vi "parse HarpMessage.vi"(13 "Round value":bool) -> (4 "HarpDataFrame":T1={"Timestamp(us)"=0.0, "Command"=16, "Error"=FALSE, "Register Address"=16, "Port"=16, "Number of Elements"=16, "Type"=16, "I8"=0, "U8"=0, "U16"=0, "I16"=0, "U32"=0, "I32"=0, "U64"=0, "I64"=0, "Float"=0.0, "U8[]"=[], "I8[]"=[], "U16[]"=[], "I16[]"=[], "U32[]"=[], "I32[]"=[], "U64[]"=[], "I64[]"=[], "Float[]"=[]} {"Timestamp(us)" format="%.6f"}, 8 "Packet Found":bool, 15 "Byte Rejected":bool)   [LabVIEW 2010]
panel:
  out "Float[]":sgl[](array[numeric])
  out "I64[]":i64[](array[numeric])
  out "U64[]":u64[](array[numeric])
  out "I32[]":i32[](array[numeric])
  out "U32[]":u32[](array[numeric])
  out "I16[]":i16[](array[numeric])
  out "U16[]":u16[](array[numeric])
  out "I8[]":i8[](array[numeric])
  out "U8[]":u8[](array[numeric])
  out "Float":sgl
  out "I64":i64
  out "U64":u64
  out "I32":i32
  out "U32":u32
  out "I16":i16
  out "U16":u16
  out "U8":u8
  out "I8":i8
  in  "Enum":T2(ring)
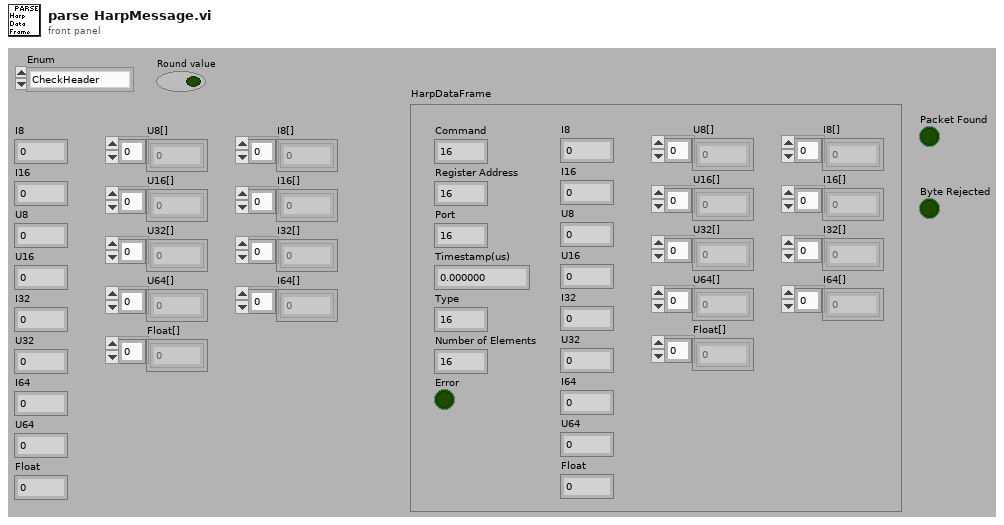
[diagram p1: front panel]
types:
  T1 = cluster{"Timestamp(us)":dbl, "Command":u8, "Error":bool, "Register Address":u8, "Port":u8, "Number of Elements":u8, "Type":u8, "I8":i8, "U8":u8, "U16":u16, "I16":i16, "U32":u32, "I32":i32, "U64":u64, "I64":i64, "Float":sgl, "U8[]":u8[], "I8[]":i8[], "U16[]":u16[], "I16[]":i16[], "U32[]":u32[], "I32[]":i32[], "U64[]":u64[], "I64[]":i64[], "Float[]":sgl[]}
  T2 = enum16{"CheckHeader", "CheckChekcum", "Parse", "Exit"}
  T3 = enum16{"CreateBuffer", "WriteBytes", "WriteByte", "AvailableMemory", "OccupiedMemory", "CheckBytes", "ReadBytes"}
  T4 = enum16{"big-endian, network order", "native, host order", "little-endian"}
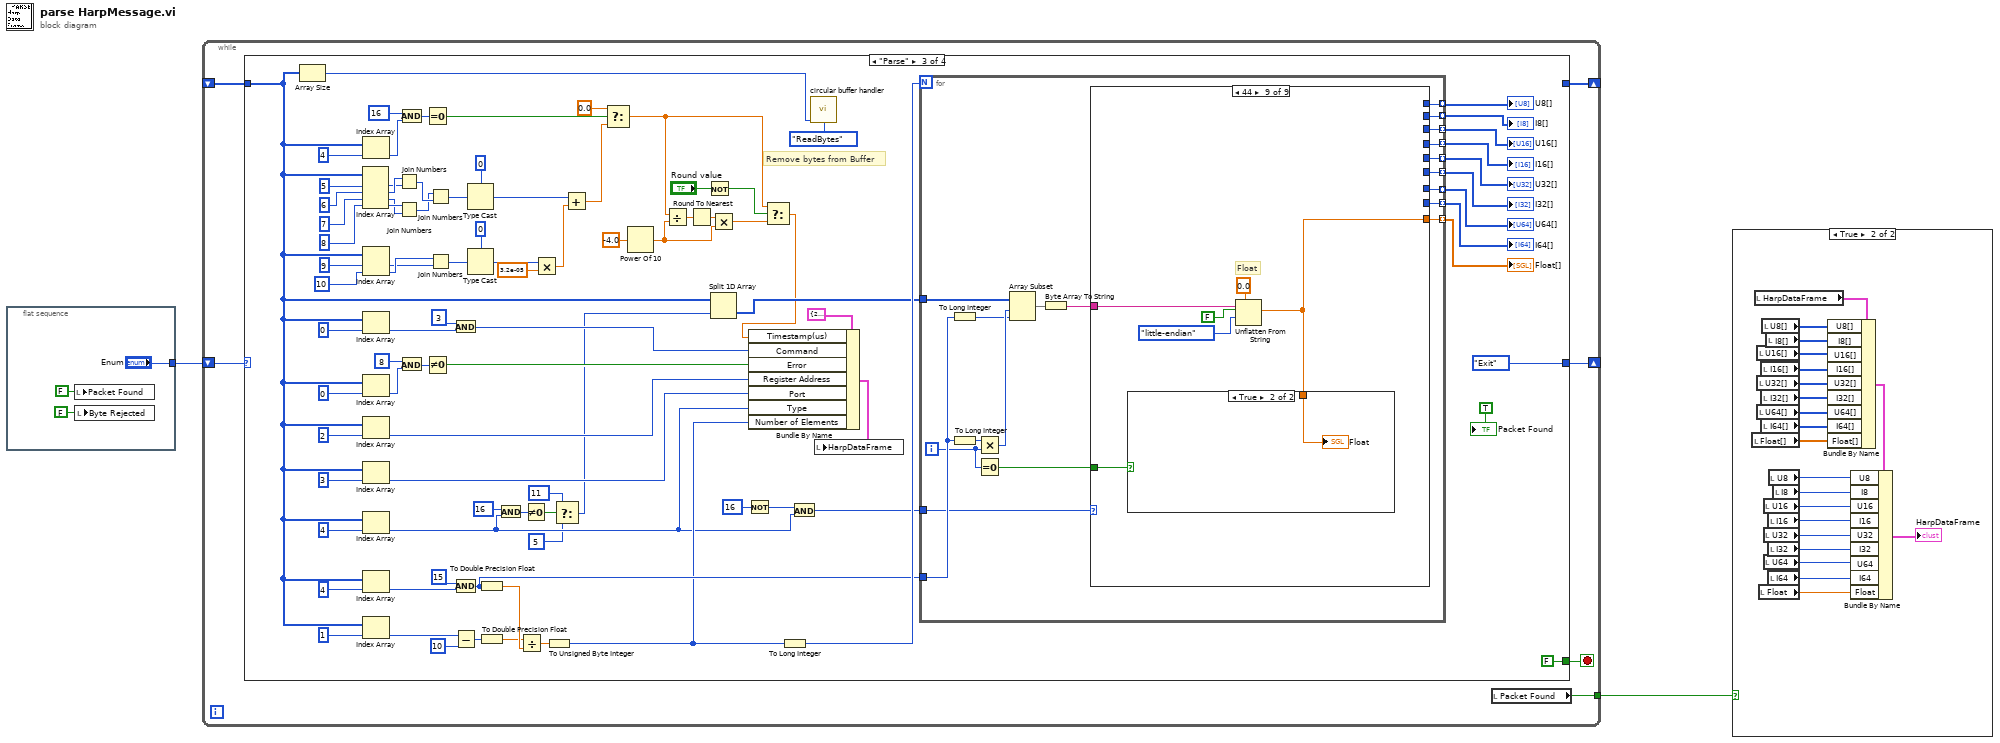
[diagram p0: block diagram]
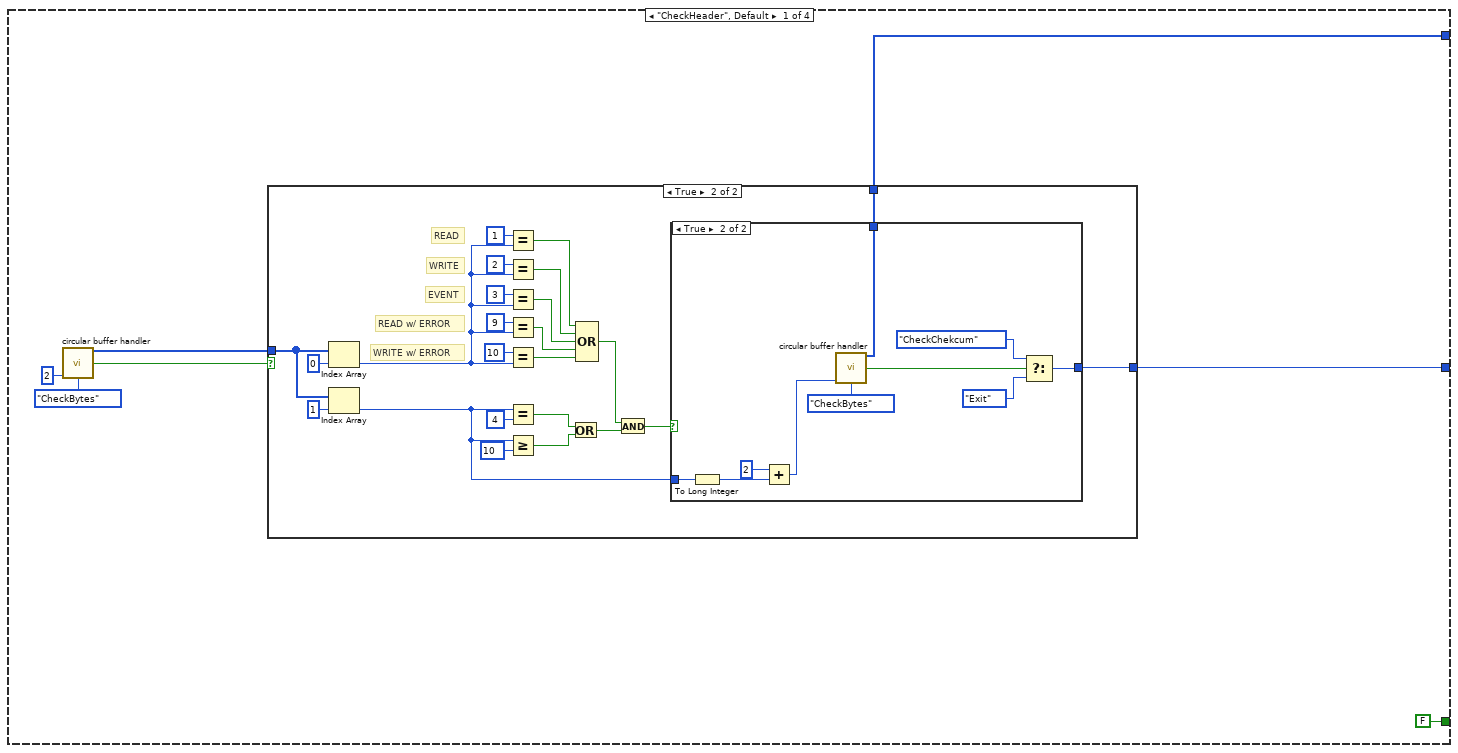
[diagram p3: hidden frame]
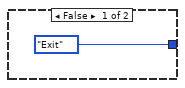
[diagram p4: hidden frame]
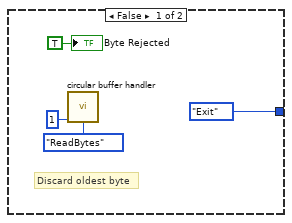
[diagram p5: hidden frame]
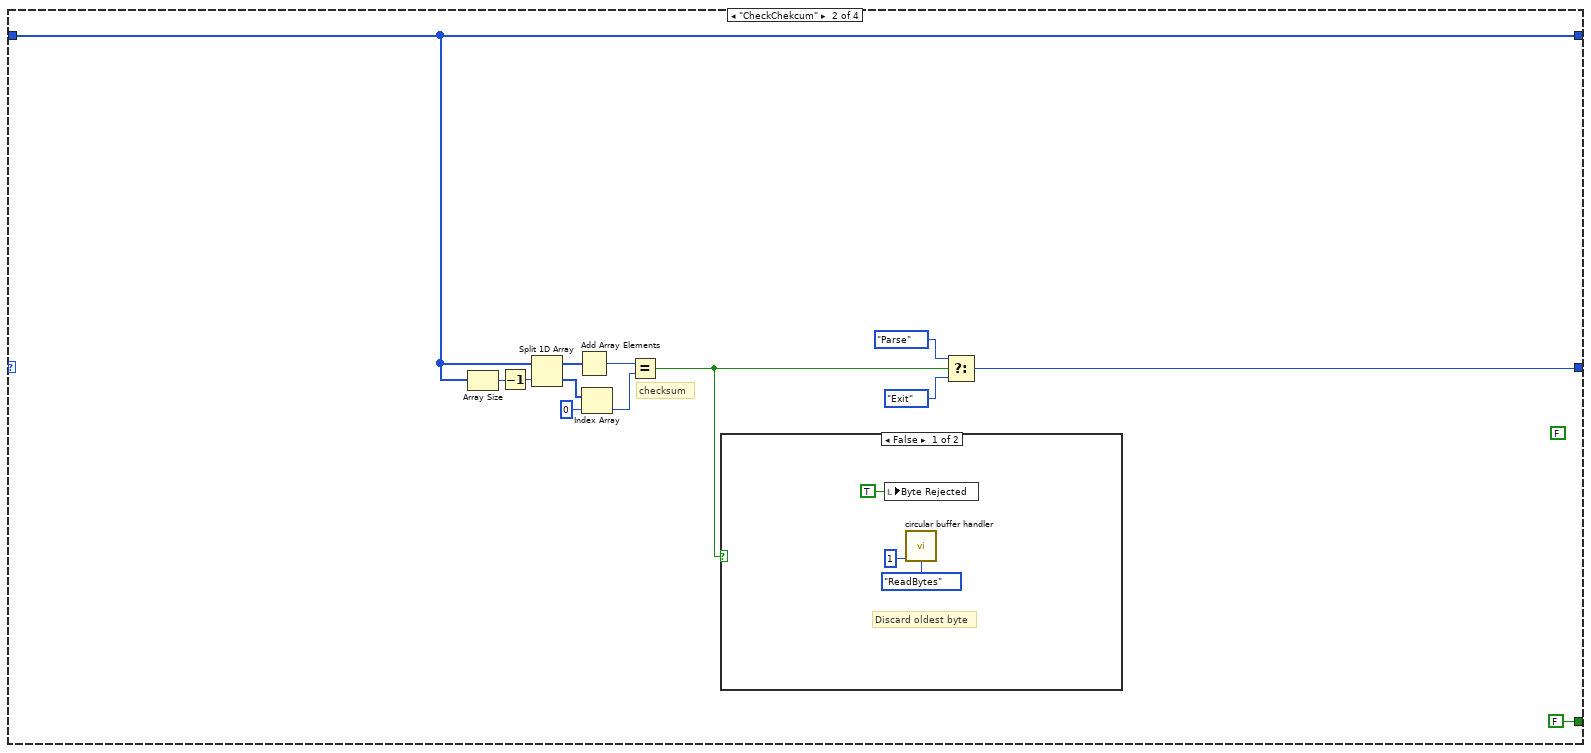
[diagram p6: hidden frame]
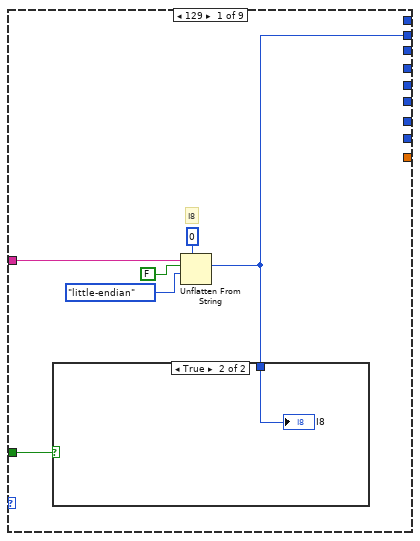
[diagram p8: hidden frame]
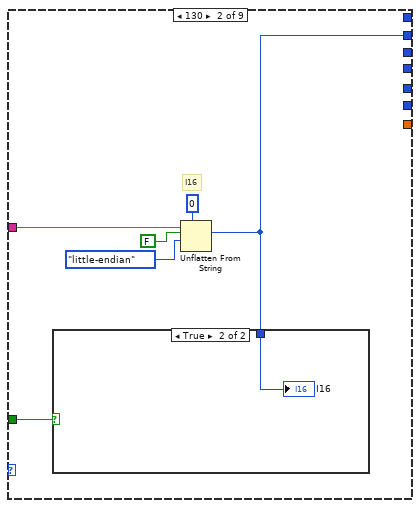
[diagram p10: hidden frame]
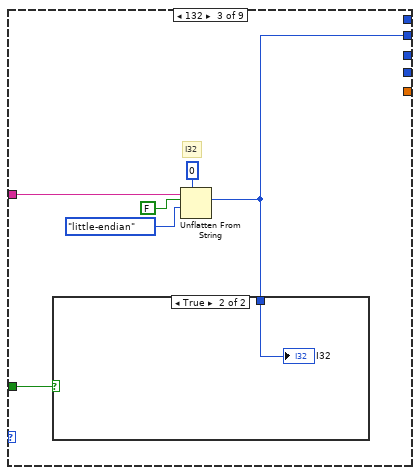
[diagram p12: hidden frame]
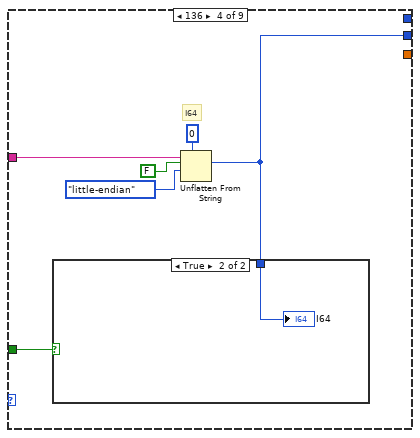
[diagram p14: hidden frame]
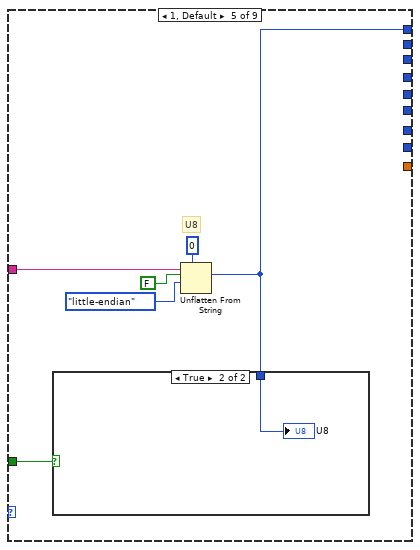
[diagram p16: hidden frame]
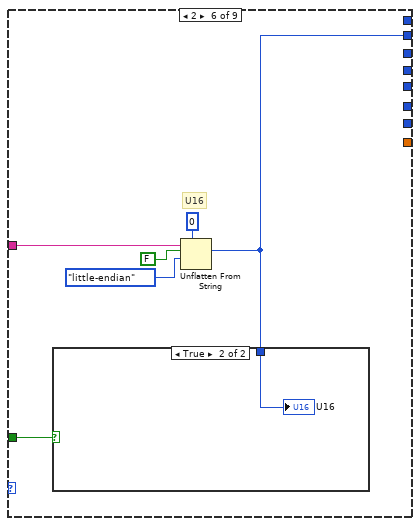
[diagram p18: hidden frame]
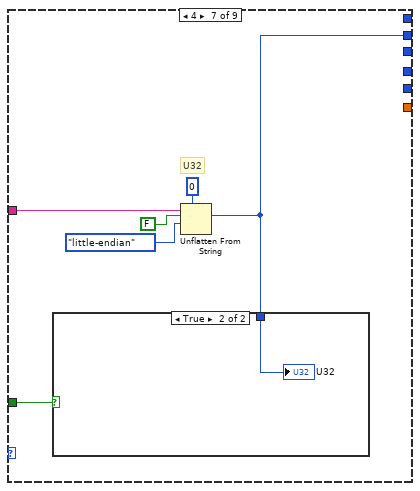
[diagram p20: hidden frame]
diagram:
  n1 = flat-sequence {
    tunnel: ["Enum"] -> w2
    frame #0 {
      n2 = local write "Packet Found"(FALSE ("PacketFound")) -> ()
      n3 = local write "Byte Rejected"(FALSE ("Byte Rejected")) -> ()
    }
  }
  n4 = while {
    shift-right: [w10] -> _
    shift-left: w2 -> [w11]
    shift-right: [w9] -> _
    shift-left: _ -> [w8]
    tunnel: [w6] -> w1
    stop <- w7 stop-if-true
    n5 = case shown="\"Parse\"" w11 {
      tunnel: [w14 w61 T2."Exit" ("Enum") T2."Exit" ("Enum")] -> w10
      tunnel: [w13 w58 _ _] -> w9
      tunnel: w8 -> [_ w58 w113 _]
      tunnel: [FALSE FALSE FALSE TRUE] -> w7
      frame "CheckHeader", Default {
        n6 = call "circular buffer handler.vi"("NumberOfBytes"=2, "Enum"=T3."CheckBytes") -> ("OutputBytes"=w15:u8[], "OK"=w16:bool)  [unwired: 11 in, 1 out]
        n7 = case shown="True" w16 {
          tunnel: w15 -> [_ w41]
          tunnel: [T2."Exit" ("Enum") w21] -> w14
          tunnel: [_ w20] -> w13
          frame False {
          }
          frame True {
            # "WRITE w/ ERROR"
            # "READ w/ ERROR"
            # "EVENT"
            # "WRITE"
            # "READ"
            n8 = Index Array(array=w41, index=0) -> (element=w35:u8)
            n9 = Index Array(array=w41, index=1) -> (element=w22:u8)
            n10 = Equal?(x=u8 1, y=w35) -> (x = y?=w34:bool)
            n11 = Equal?(x=u8 2, y=w35) -> (x = y?=w33:bool)
            n12 = Equal?(x=u8 3, y=w35) -> (x = y?=w32:bool)
            n13 = Equal?(x=u8 9, y=w35) -> (x = y?=w31:bool)
            n14 = Equal?(x=u8 10, y=w35) -> (x = y?=w30:bool)
            n15 = Equal?(x=w22, y=u8 4 ("x")) -> (x = y?=w27:bool)
            n16 = Greater Or Equal?(x=w22, y=u8 10 ("x")) -> (x >= y?=w26:bool)
            n17 = Or(x=w27, y=w26) -> (x .or. y?=w25:bool)
            n18 = Compound Arithmetic op=OR(w34, w33, w32, w31, w30) -> (w24:bool)
            n19 = And(x=w24, y=w25) -> (x .and. y?=w23:bool)
            n20 = case shown="True" w23 {
              tunnel: w22 -> [_ w56]
              tunnel: [T2."Exit" ("Enum") w53] -> w21
              tunnel: [_ w48] -> w20
              frame False {
                # "Discard oldest byte"
                n21 = call "circular buffer handler.vi"("NumberOfBytes"=1, "Enum"=T3."ReadBytes") -> ()  [unwired: 11 in, 3 out]
                "Byte Rejected" <- TRUE ("PacketFound")
              }
              frame True {
                n22 = To Long Integer(number=w56) -> (32bit integer=w54:i32)
                n23 = Add(x=2, y=w54) -> (x+y=w50:i32)
                n24 = call "circular buffer handler.vi"("NumberOfBytes"=w50, "Enum"=T3."CheckBytes") -> ("OutputBytes"=w48:u8[], "OK"=w49:bool)  [unwired: 11 in, 1 out]
                n25 = Select(t=T2."CheckChekcum" ("Enum"), s=w49, f=T2."Exit" ("Enum")) -> (s? t:f=w53:T2)
              }
            }
          }
        }
      }
      frame "CheckChekcum" {
        (unwired) FALSE ("PacketFound")
        # "checksum"
        n26 = Array Size(array=w58) -> (size(s)=w70:i32)
        n27 = Decrement(x=w70) -> (x-1=w69:i32)
        n28 = Split 1D Array(array=w58, index=w69) -> (first subarray=w65:u8[], second subarray=w66:u8[])
        n29 = Add Array Elements(numeric array=w65) -> (sum=w68:u8)
        n30 = Index Array(array=w66, index=0) -> (element=w64:u8)
        n31 = Equal?(x=w68, y=w64) -> (x = y?=w59:bool)
        n32 = case shown="False" w59 {
          frame False {
            # "Discard oldest byte"
            n33 = local write "Byte Rejected"(TRUE ("Byte Rejected")) -> ()
            n34 = call "circular buffer handler.vi"("NumberOfBytes"=1, "Enum"=T3."ReadBytes") -> ()  [unwired: 11 in, 3 out]
          }
          frame True {
          }
        }
        n35 = Select(t=T2."Parse" ("Enum"), s=w59, f=T2."Exit" ("Enum")) -> (s? t:f=w61:T2)
      }
      frame "Parse" {
        # "Remove bytes from Buffer"
        n36 = Array Size(array=w113) -> (size(s)=w115:i32)
        n37 = Index Array(array=w113, index #1=5 ("index"), index #2=6 ("index"), index #3=7 ("index"), index #4=8 ("index")) -> (element #1=w155:u8, element #2=w159:u8, element #3=w156:u8, element #4=w157:u8)
        n38 = Index Array(array=w113, index=4) -> (element=w140:u8)
        n39 = Index Array(array=w113, index #1=9 ("index"), index #2=10 ("index")) -> (element #1=w144:u8, element #2=w145:u8)
        n40 = Index Array(array=w113, index=0) -> (element=w134:u8)
        n41 = Index Array(array=w113, index=0) -> (element=w133:u8)
        n42 = Index Array(array=w113, index=2) -> (element=w99:u8)
        n43 = Index Array(array=w113, index=3) -> (element=w98:u8)
        n44 = Index Array(array=w113, index=4) -> (element=w89:u8)
        n45 = Index Array(array=w113, index=4) -> (element=w126:u8)
        n46 = Index Array(array=w113, index=1) -> (element=w122:u8)
        n47 = Join Numbers(hi=w159, lo=w155) -> ((hi.lo)=w160:u16)
        n48 = Join Numbers(hi=w157, lo=w156) -> ((hi.lo)=w158:u16)
        n49 = And(x=u8 16, y=w140) -> (x .and. y?=w164:u8)
        n50 = And(x=u8 8, y=w133) -> (x .and. y?=w131:u8)
        n51 = Equal To 0?(x=w164) -> (x = 0?=w139:bool)
        n52 = Not Equal To 0?(x=w131) -> (x != 0?=w100:bool)
        n53 = Join Numbers(hi=w158, lo=w160) -> ((hi.lo)=w150:u32)
        n54 = Join Numbers(hi=w145, lo=w144) -> ((hi.lo)=w146:u16)
        n55 = And(x=u8 3, y=w134) -> (x .and. y?=w101:u8)
        n56 = And(x=u8 15, y=w126) -> (x .and. y?=w111:u8)
        n57 = Subtract(x=w122, y=u8 10) -> (x-y=w120:u8)
        n58 = Type Cast(type=u32 0 ("byte count"), x=w150) -> (*(type *) &x=w162:u32)
        n59 = Type Cast(type=u16 0 ("byte count"), x=w146) -> (*(type *) &x=w148:u16)
        n60 = To Double Precision Float(number=w111) -> (double precision float=w118:dbl)
        n61 = To Double Precision Float(number=w120) -> (double precision float=w117:dbl)
        n62 = And(x=u8 16, y=w89) -> (x .and. y?=w90:u8)
        n63 = Divide(x=w117, y=w118) -> (x/y=w119:dbl)
        n64 = Not Equal To 0?(x=w90) -> (x != 0?=w88:bool)
        n65 = Multiply(x=w148, y=3.2e-05) -> (x*y=w163:dbl)
        n66 = To Unsigned Byte Integer(number=w119) -> (unsigned 8bit integer=w97:u8)
        n67 = Select(t=u8 11, s=w88, f=u8 5) -> (s? t:f=w85:u8)
        n68 = Add(x=w162, y=w163) -> (x+y=w138:dbl)
        n69 = Select(t=0.0, s=w139, f=w138) -> (s? t:f=w77:dbl)
        n70 = Power Of 10(x=-4.0) -> (10^x=w80:dbl)
        n71 = Divide(x=w77, y=w80) -> (x/y=w82:dbl)
        n72 = Round To Nearest(number=w82) -> (nearest integer value=w81:dbl)
        n73 = Not(x="Round value") -> (.not. x?=w74:bool)
        n74 = Multiply(x=w81, y=w80) -> (x*y=w78:dbl)
        n75 = Split 1D Array(array=w113, index=w85) -> (second subarray=w92:u8[])  [unwired: 1 out]
        n76 = Not(x=u8 16) -> (.not. x?=w95:u8)
        n77 = Select(t=w77, s=w74, f=w78) -> (s? t:f=w76:dbl)
        n78 = Bundle By Name(cluster=T1 {"Timestamp(us)"=2218.246816, "Command"=1, "Error"=FALSE, "Register Address"=18, "Port"=255, "Number of Elements"=1, "Type"=84, "I8"=0, "U8"=0, "U16"=0, "I16"=0, "U32"=0, "I32"=0, "U64"=0, "I64"=0, "Float"=0.0, "U8[]"=[0], "I8[]"=[0], "U16[]"=[0], "I16[]"=[0], "U32[]"=[0], "I32[]"=[0], "U64[]"=[0], "I64[]"=[0], "Float[]"=[0.0]} ("HarpDataFrame"), "Timestamp(us)"=w76, "Command"=w101, "Error"=w100, "Register Address"=w99, "Port"=w98, "Type"=w89, "Number of Elements"=w97) -> (w84:T1)
        n79 = To Long Integer(number=w97) -> (32bit integer=w112:i32)
        n80 = And(x=w95, y=w89) -> (x .and. y?=w93:u8)
        n81 = call "circular buffer handler.vi"("NumberOfBytes"=w115, "Enum"=T3."ReadBytes") -> ()  [unwired: 11 in, 3 out]
        n82 = local write "HarpDataFrame"(w84) -> ()
        n83 = for {
          N: w112 -> [_]
          tunnel: w92 -> [w183]
          tunnel: w111 -> [w182]
          tunnel: w93 -> [w178]
          tunnel: [w175] -> w110 mode=indexing
          tunnel: [w174] -> w109 mode=indexing
          tunnel: [w173] -> w108 mode=indexing
          tunnel: [w172] -> w107 mode=indexing
          tunnel: [w171] -> w106 mode=indexing
          tunnel: [w170] -> w105 mode=indexing
          tunnel: [w169] -> w104 mode=indexing
          tunnel: [w168] -> w102 mode=indexing
          tunnel: [w167] -> w103 mode=indexing
          i -> [w177]
          n84 = To Long Integer(number=w182) -> (32bit integer=w179:i32)
          n85 = To Long Integer(number=w182) -> (32bit integer=w180:i32)
          n86 = Multiply(x=w180, y=w177) -> (x*y=w181:i32)
          n87 = Equal To 0?(x=w177) -> (x = 0?=w176:bool)
          n88 = Array Subset(array=w183, index=w181, length=w179) -> (w184:u8[])
          n89 = Byte Array To String(unsigned byte array=w184) -> (string=w185:string)
          n90 = case shown="44" w178 {
            tunnel: w185 -> [w190 w197 w204 w211 w218 w225 w232 w239 w246]
            tunnel: w176 -> [w187 w194 w201 w208 w215 w222 w229 w236 w243]
            tunnel: [_ _ _ _ w214 _ _ _ _] -> w175
            tunnel: [w186 _ _ _ _ _ _ _ _] -> w174
            tunnel: [_ _ _ _ _ w221 _ _ _] -> w173
            tunnel: [_ w193 _ _ _ _ _ _ _] -> w172
            tunnel: [_ _ _ _ _ _ w228 _ _] -> w171
            tunnel: [_ _ w200 _ _ _ _ _ _] -> w170
            tunnel: [_ _ _ _ _ _ _ w235 _] -> w169
            tunnel: [_ _ _ w207 _ _ _ _ _] -> w168
            tunnel: [_ _ _ _ _ _ _ _ w242] -> w167
            frame 129 {
              # "I8"
              n91 = Unflatten From String(type=i8 0 ("Port"), binary string=w190, data includes array or string size? (T)=FALSE, byte order (0:big-endian, network order)=T4."little-endian") -> (value=w186:i8)  [unwired: 1 in, 2 out]
              n92 = case shown="True" w187 {
                tunnel: w186 -> [_ w192]
                frame False {
                }
                frame True {
                  "I8" <- w192
                }
              }
            }
            frame 130 {
              # "I16"
              n93 = Unflatten From String(type=i16 0 ("Port"), binary string=w197, data includes array or string size? (T)=FALSE, byte order (0:big-endian, network order)=T4."little-endian") -> (value=w193:i16)  [unwired: 1 in, 2 out]
              n94 = case shown="True" w194 {
                tunnel: w193 -> [_ w199]
                frame False {
                }
                frame True {
                  "I16" <- w199
                }
              }
            }
            frame 132 {
              # "I32"
              n95 = Unflatten From String(type=0 ("Port"), binary string=w204, data includes array or string size? (T)=FALSE, byte order (0:big-endian, network order)=T4."little-endian") -> (value=w200:i32)  [unwired: 1 in, 2 out]
              n96 = case shown="True" w201 {
                tunnel: w200 -> [_ w206]
                frame False {
                }
                frame True {
                  "I32" <- w206
                }
              }
            }
            frame 136 {
              # "I64"
              n97 = Unflatten From String(type=i64 0 ("Port"), binary string=w211, data includes array or string size? (T)=FALSE, byte order (0:big-endian, network order)=T4."little-endian") -> (value=w207:i64)  [unwired: 1 in, 2 out]
              n98 = case shown="True" w208 {
                tunnel: w207 -> [_ w213]
                frame False {
                }
                frame True {
                  "I64" <- w213
                }
              }
            }
            frame 1, Default {
              # "U8"
              n99 = Unflatten From String(type=u8 0 ("Port"), binary string=w218, data includes array or string size? (T)=FALSE, byte order (0:big-endian, network order)=T4."little-endian") -> (value=w214:u8)  [unwired: 1 in, 2 out]
              n100 = case shown="True" w215 {
                tunnel: w214 -> [_ w220]
                frame False {
                }
                frame True {
                  "U8" <- w220
                }
              }
            }
            frame 2 {
              # "U16"
              n101 = Unflatten From String(type=u16 0 ("Port"), binary string=w225, data includes array or string size? (T)=FALSE, byte order (0:big-endian, network order)=T4."little-endian") -> (value=w221:u16)  [unwired: 1 in, 2 out]
              n102 = case shown="True" w222 {
                tunnel: w221 -> [_ w227]
                frame False {
                }
                frame True {
                  "U16" <- w227
                }
              }
            }
            frame 4 {
              # "U32"
              n103 = Unflatten From String(type=u32 0 ("Port"), binary string=w232, data includes array or string size? (T)=FALSE, byte order (0:big-endian, network order)=T4."little-endian") -> (value=w228:u32)  [unwired: 1 in, 2 out]
              n104 = case shown="True" w229 {
                tunnel: w228 -> [_ w234]
                frame False {
                }
                frame True {
                  "U32" <- w234
                }
              }
            }
            frame 8 {
              # "U64"
              n105 = Unflatten From String(type=u64 0 ("Port"), binary string=w239, data includes array or string size? (T)=FALSE, byte order (0:big-endian, network order)=T4."little-endian") -> (value=w235:u64)  [unwired: 1 in, 2 out]
              n106 = case shown="True" w236 {
                tunnel: w235 -> [_ w241]
                frame False {
                }
                frame True {
                  "U64" <- w241
                }
              }
            }
            frame 68 {
              # "Float"
              n107 = Unflatten From String(type=sgl 0.0 ("Port"), binary string=w246, data includes array or string size? (T)=FALSE, byte order (0:big-endian, network order)=T4."little-endian") -> (value=w242:sgl)  [unwired: 1 in, 2 out]
              n108 = case shown="True" w243 {
                tunnel: w242 -> [_ w248]
                frame False {
                }
                frame True {
                  "Float" <- w248
                }
              }
            }
          }
        }
        "U8[]" <- w110
        "I8[]" <- w109
        "U16[]" <- w108
        "I16[]" <- w107
        "U32[]" <- w106
        "I32[]" <- w105
        "U64[]" <- w104
        "I64[]" <- w102
        "Float[]" <- w103
        "Packet Found" <- TRUE ("PacketFound")
      }
      frame "Exit" {
        (unwired) FALSE ("PacketFound")
      }
    }
    n109 = local read "Packet Found"() -> (w6:bool)
  }
  n110 = case shown="True" w1 {
    frame False {
    }
    frame True {
      n111 = local read "Float[]"() -> (w263:sgl[])
      n112 = local read "HarpDataFrame"() -> (w252:T1)
      n113 = local read "U16[]"() -> (w269:u16[])
      n114 = local read "U32[]"() -> (w267:u32[])
      n115 = local read "U64[]"() -> (w265:u64[])
      n116 = local read "Float"() -> (w253:sgl)
      n117 = local read "I16[]"() -> (w268:i16[])
      n118 = local read "I32[]"() -> (w266:i32[])
      n119 = local read "I64[]"() -> (w264:i64[])
      n120 = local read "U8[]"() -> (w271:u8[])
      n121 = local read "U16"() -> (w259:u16)
      n122 = local read "U32"() -> (w257:u32)
      n123 = local read "U64"() -> (w255:u64)
      n124 = local read "I8[]"() -> (w270:i8[])
      n125 = local read "I16"() -> (w258:i16)
      n126 = local read "I32"() -> (w256:i32)
      n127 = local read "I64"() -> (w254:i64)
      n128 = local read "U8"() -> (w261:u8)
      n129 = local read "I8"() -> (w260:i8)
      n130 = Bundle By Name(cluster=w252, "U8[]"=w271, "I8[]"=w270, "U16[]"=w269, "I16[]"=w268, "U32[]"=w267, "I32[]"=w266, "U64[]"=w265, "I64[]"=w264, "Float[]"=w263) -> (w262:T1)
      n131 = Bundle By Name(cluster=w262, "U8"=w261, "I8"=w260, "U16"=w259, "I16"=w258, "U32"=w257, "I32"=w256, "U64"=w255, "I64"=w254, "Float"=w253) -> (→"HarpDataFrame":T1)
    }
  }
